vi "main.vi"(0 "Test Pins":T7, 1 "Caller Information":T8, 5 "Test Inputs":T12={"Load Current in A"=0.0, "Input Voltage in V"=[], "Nominal Output Voltage in V"=0.0, "Advance Setting"={"Prepare"={"Load SMU Output Function"=enum."VoltageSource"}, "Stimulus And Measure"={"Loop Delay in milliSecond"=1}}}, 11 "error in":errorcluster) -> (4 "Test Results":T11 {"Line Regulation in %" format="%#.5g"; "Input Voltage in V" format="%#.5g"; "Input Current in A" format="%#.5g"; "Load Current in A" format="%#.5g"; "Output Voltage in V" format="%#.5g"}, 15 "error out":errorcluster)   [LabVIEW 2020, in "LDO Line Regulation.lvlib"]
doc: "<b>Caller</b> Information is input for framework components. Mode should be set to <b>Automation</b> when running from TestStand. Sequence Context should be set to <b>ThisContext</b> when running from TestStand. The values will be updated everytime the setting is applied using \"Edit\" dialog.\n\n<b>Test Pins</b> is names of pins available in the pinmap file. Provide the right pins for the required functionality.\n\n<b>Test Inputs</b> is input required for the measurement to perform.\n\n<b>error in</b> is meant for the sequencing. <b>error in</b> should be <b>no error</b> always.\n\n<b>Test Results</b> contains all the measured data during the measurement and processed results.\n\n<b>error out</b> contains the error occured during measurement.\n\nCheck measurement documentation for more information (<Program Files>\\Soliton Technologies\\MeasurementSuite\\CodeModules\\LDO\\LDO Line Regulation.pdf)"
uses:
  LDO Line Regulation.lvlib
  Typedefs/Test Results.ctl
  Typedefs/Test Inputs.ctl
  Typedefs/Advance Settings.ctl
  Reusables/Instrument APIs/Load Output Function.ctl
  <userlib>/_Soliton/Measurement Suite/Reusables/Plugin Common/Typedefs/Caller Events.ctl
  <userlib>/_Soliton/Measurement Suite/Reusables/Plugin Common/Typedefs/Caller Information.ctl
  <userlib>/_Soliton/Measurement Suite/Reusables/Plugin Common/Typedefs/Caller Mode.ctl
  Typedefs/Test Pins.ctl
  Typedefs/Pin Dropdown.ctl
  <userlib>/_Soliton/Measurement Suite/Reusables/Plugin Common/Typedefs/Termination Monitor Info.ctl
  <vilib>/Utility/error.llb/DialogType.ctl
  dc46d5cc-eb00-4f7e-b59b-e7fbb9f2ed4c.vi
  f0cc231b-6294-4813-9d5b-a7ddc5043ff2.vi
  f8cfc4b9-01f6-4b8f-8ca0-5ef2fe22dc8a.vi
  be024a05-4f6c-4aec-bf2b-5f4e194505bf.vi
  d9360132-6dee-4b9e-876e-39170c807331.vi
  f5d431a0-41a8-4d91-8ed4-f3030fcb2f72.vi
  1f043610-9790-4767-a48a-a9d4642a4a56.vi
  bb3e62c4-a2c2-4505-9438-f842dd651d6c.vi
  ce2ee1e5-697c-4608-b941-8c9b0f21ffd9.vi
  3fc05b7f-d306-4c90-81fb-acd80905c629.vi
  34057e1b-ed15-48f4-a73e-55eccb727778.vi
  <userlib>/_Soliton/Measurement Suite/Reusables/InstrumentSessionAPIs/SessionManagerApiPath.vi
  <vilib>/Utility/sysdir.llb/Get System Directory.vi
  <vilib>/Utility/LVLibp/Get Exported File Path.vi
  <userlib>/_Soliton/Measurement Suite/Reusables/Errors/Error 6001.vi
  <userlib>/_Soliton/Measurement Suite/Reusables/Plugin Common/Plugin Common.lvlib
  <userlib>/_Soliton/Measurement Suite/Reusables/Queue Driver/Plugin Queue Driver.lvlib
panel:
  out "Progress":i32(slide) scale=-1.0..5.0
  in  "Terminate":bool
  in  "Run":bool caption="Measure"
  in  "Exit":bool
  out "Header":string
  in  "Tab Enum":T1(radio)
  out "Tab Control":T2(tab)
  in  "SystemSetup":T4={"Set Input Voltage"={"PinStatus"=0, "PinName"="", "Info"=TRUE}, "Measure Input Voltage"={"PinStatus"=0, "PinName"="", "Info"=TRUE}, "Measure Input Current"={"PinStatus"=0, "PinName"="", "Info"=TRUE}, "Set Load Current"={"PinStatus"=0, "PinName"="", "Info"=TRUE}, "Measure Output Voltage"={"PinStatus"=0, "PinName"="", "Info"=TRUE}, "Measure Load Current"={"PinStatus"=0, "PinName"="", "Info"=TRUE}}
  in  "Step Input":T5 {"Step Size (V)" min=0.0 format="%#_6p"; "Stop Value (V)" format="%#_6p"; "Start Value (V)" format="%#_6p"}
  in  "Customize Sweep Value":bool
  in  "Input Voltage (V)":dbl[](array[numeric]) format="%#_6p"
  in  "Nominal Output Voltage (V)":dbl format="%#_6p"
  in  "Customize Sweep Value":enum32{"Item 0", "Item 1"}(radio)
  in  "Load Current (A)":dbl format="%#_6p"
  in  "Advanced Settings":bool
  out "Result Tab":T6(tab)
  out "Line Regulation":cluster{"Iload (mA)":dbl[], "Vout (V)":dbl[]}(graph)
  out "Measured Values":string[][](table)
  out "Line Regulation (%/V)":dbl format="%#.3g"
  in  "Result Enum":T6(radio)
  out "Line Regulation (%)":dbl format="%#.3g"
  in  "DataLogPath":path
  in  "Caller Events":T10
  in  "ErrorOccured":errorcluster
  # "Supports NIDmmInstrument"
  # "Supports NIDmmInstrument"
  # "Supports NIDCPowerInstrument"
  # "Supports NIDCPowerInstrument"
  # "Supports NIDCPowerInstrument"
  # "Supports NIDCPowerInstrument"
  # "Fill Input Voltage list using the following"
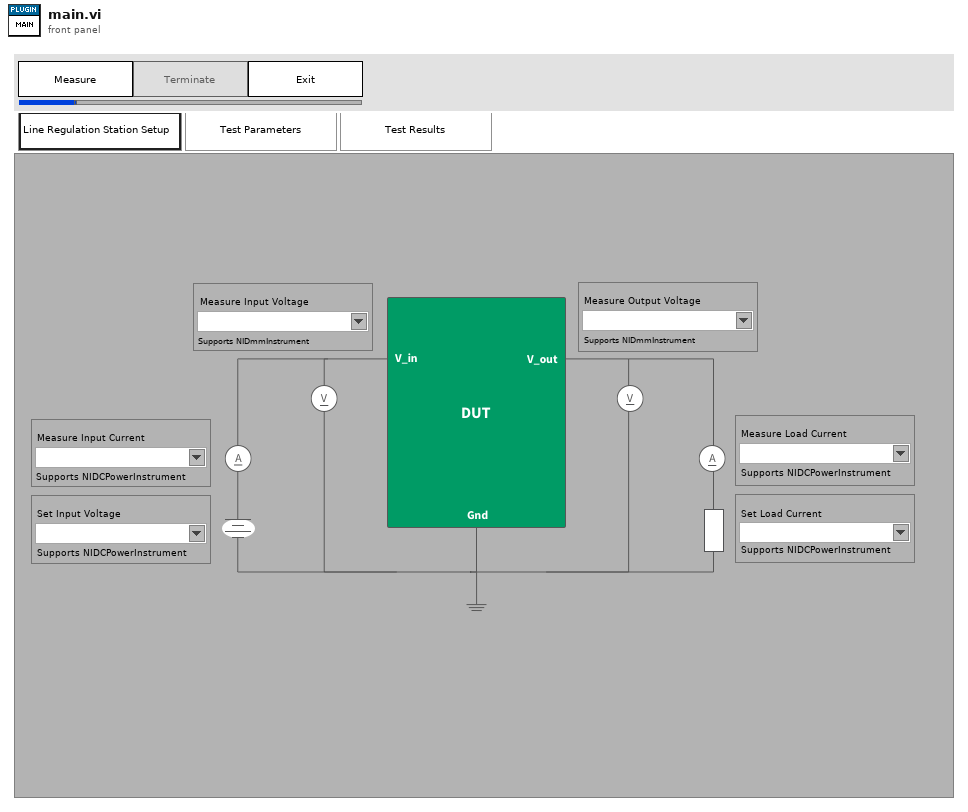
[diagram p1: front panel]
types:
  T1 = enum32{"Station Setup", "Test Parameters", "Test Results"}
  T2 = enum32{"Station Setup", "Test Parameters", "Test Results", "Debug"}
  T3 = typedef "LDO Line Regulation.lvlib/Pin Dropdown.ctl" = cluster{"PinStatus":u16, "PinName":string, "Info":bool}
  T4 = cluster{"Set Input Voltage":T3, "Measure Input Voltage":T3, "Measure Input Current":T3, "Set Load Current":T3, "Measure Output Voltage":T3, "Measure Load Current":T3}
  T5 = cluster{"Start Value (V)":dbl, "Stop Value (V)":dbl, "Step Size (V)":dbl}
  T6 = enum32{"Line Regulation Curve", "Measured Value Table View"}
  T7 = typedef "LDO Line Regulation.lvlib/Test Pins.ctl" = cluster{"Set Input Voltage":string, "Measure Input Voltage":string, "Measure Input Current":string, "Set Load Current":string, "Measure Output Voltage":string, "Measure Load Current":string}
  T8 = typedef "Plugin Common.lvlib/Caller Information.ctl" = cluster{"Mode":T9, "Sequence Context":refnum<k7>}
  T9 = typedef "Caller Mode.ctl" = enum16{"Standalone", "Automation", "MeasurementSuite"}
  T10 = typedef "Plugin Common.lvlib/Caller Events.ctl" = cluster{"Caller Event":refnum<user-event>}
  T11 = typedef "LDO Line Regulation.lvlib/Test Results.ctl" = cluster{"Input Voltage in V":dbl[], "Input Current in A":dbl[], "Output Voltage in V":dbl[], "Load Current in A":dbl[], "Line Regulation in %/V":dbl, "Line Regulation in %":dbl}
  T12 = typedef "LDO Line Regulation.lvlib/Test Inputs.ctl" = cluster{"Load Current in A":dbl, "Input Voltage in V":dbl[], "Nominal Output Voltage in V":dbl, "Advance Setting":T13}
  T13 = typedef "LDO Line Regulation.lvlib/Advance Settings.ctl" = cluster{"Prepare":cluster{"Load SMU Output Function":T14}, "Stimulus And Measure":cluster{"Loop Delay in milliSecond":u32}}
  T14 = typedef "Load Output Function.ctl" = enum16{"VoltageSource", "CurrentSource"}
  T15 = typedef "Plugin Common.lvlib/Termination Monitor Info.ctl" = cluster{"Caller Information":T8, "Execution":refnum<k7>, "Termination Monitor":refnum<k7>, "Type":string, "Plugin Name":string}
  T16 = cluster{"Termination Monitor Info":T15, "Test Inputs":T12, "Test Results":T11, "Test Results[][]":string[][], "Test Pins":T7, "Logger Folder Path":path, "Valid Logger Path?":bool, "Logger File Path":path, "UI Ctls":refnum<vi>[]}
  T17 = enum8{"Enabled", "Disabled", "Disabled and Grayed Out"}
  T18 = cluster{"Start Value":dbl, "Stop Value":dbl, "Step Size":dbl}
  T19 = cluster{"Input Voltage in V":dbl[], "Output Voltage in V":dbl[]}
  T20 = typedef "DialogType.ctl" = u16
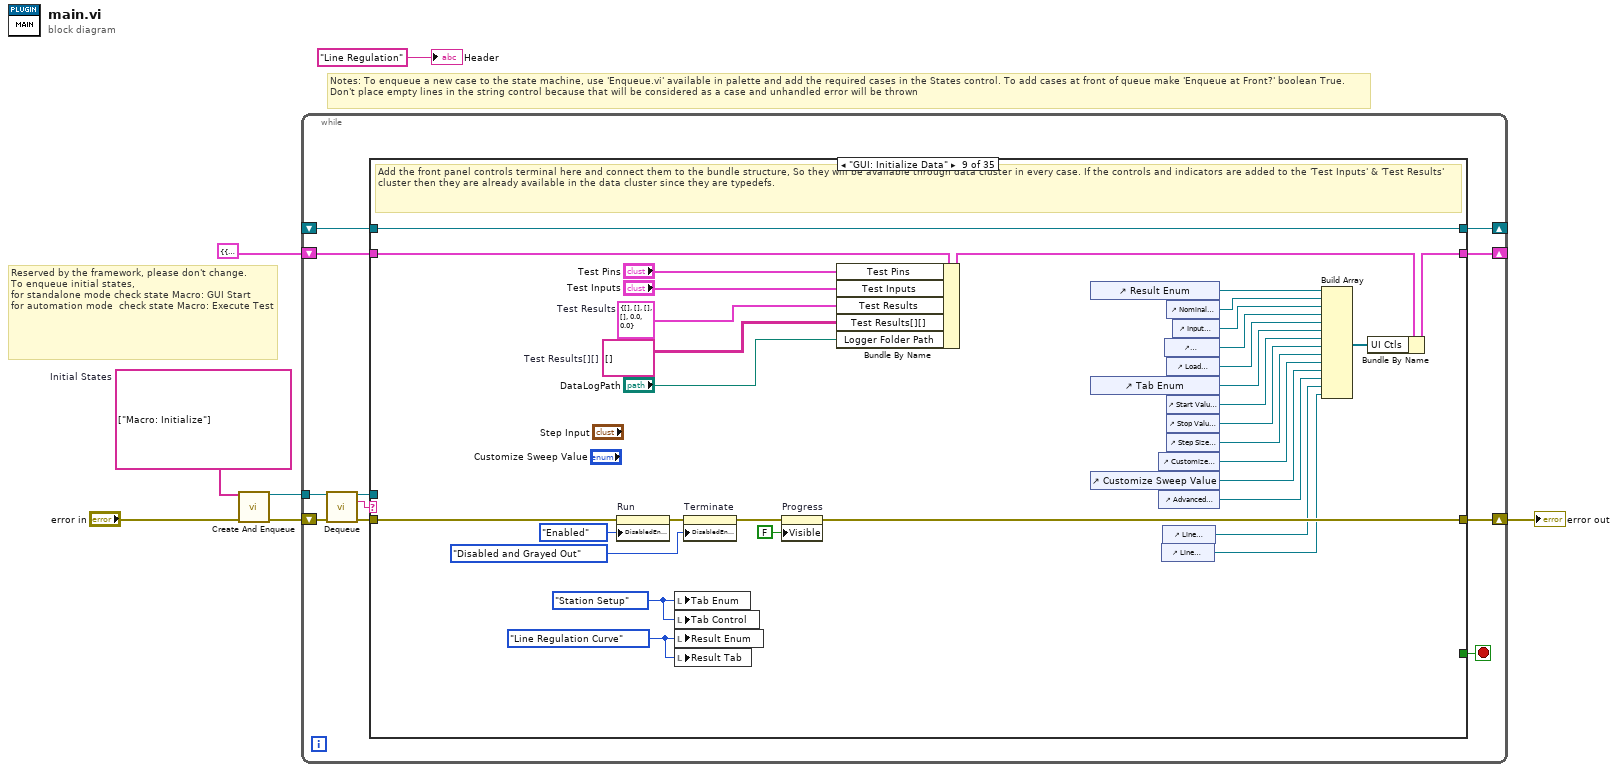
[diagram p0: block diagram]
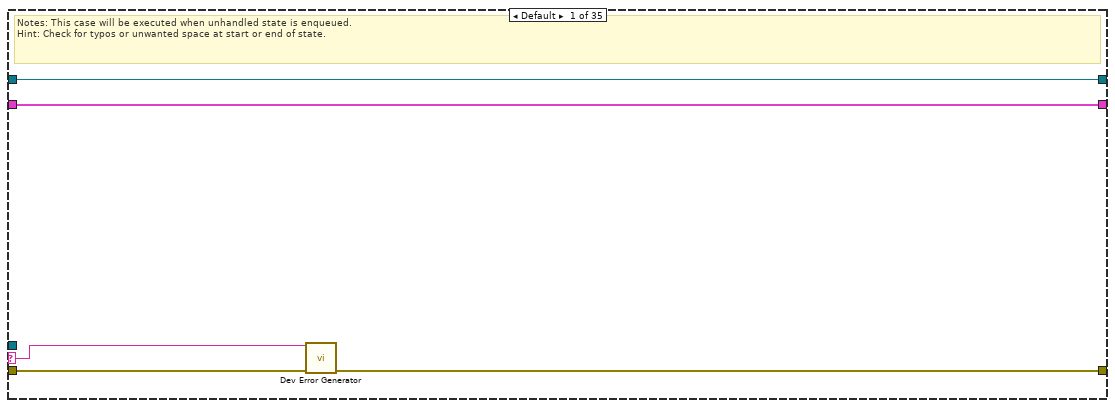
[diagram p2: hidden frame]
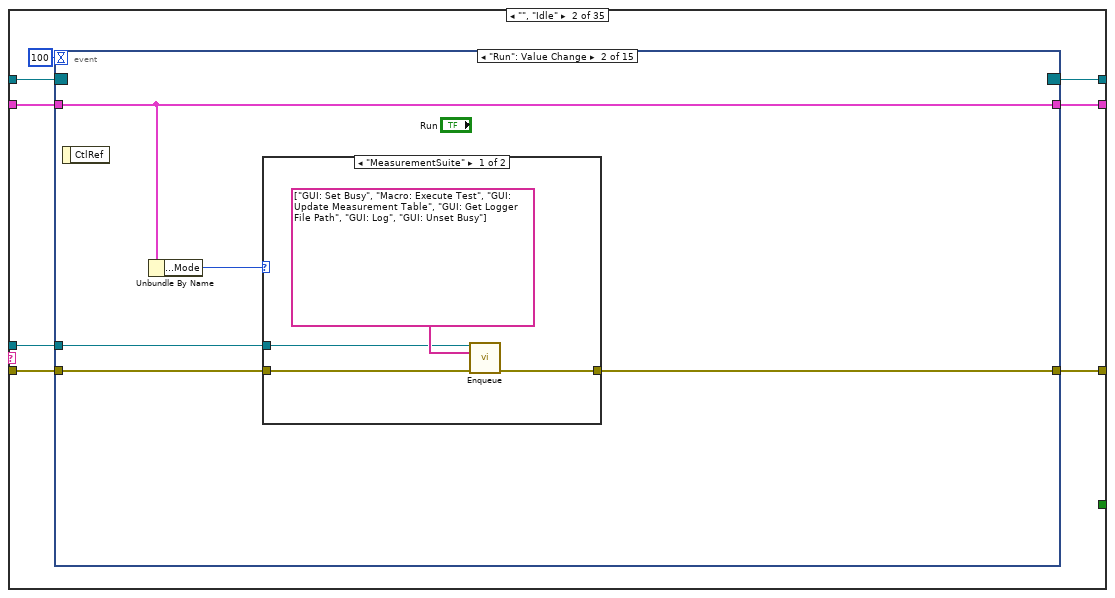
[diagram p3: hidden frame]
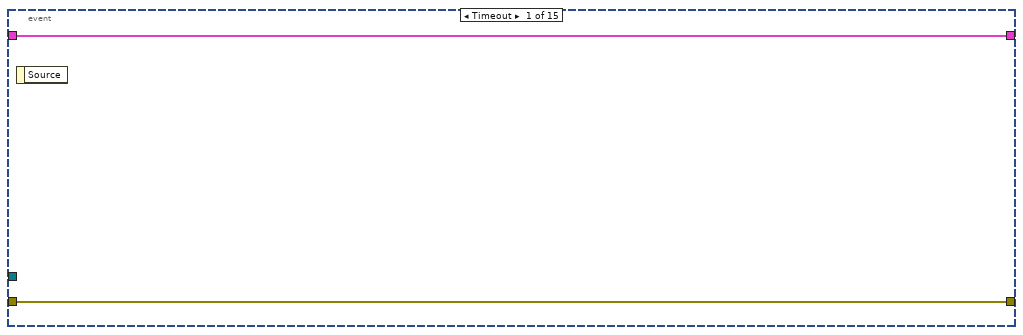
[diagram p4: hidden frame]
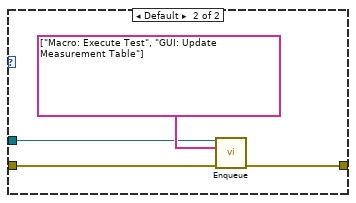
[diagram p5: hidden frame]
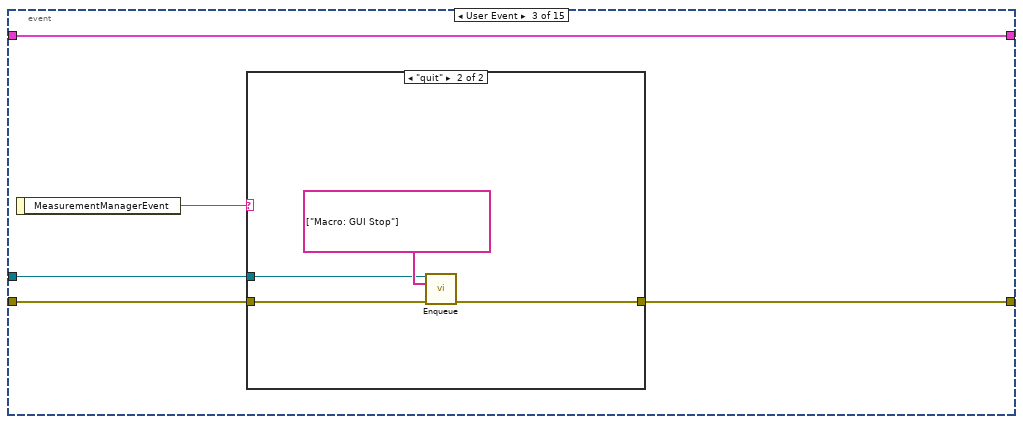
[diagram p6: hidden frame]
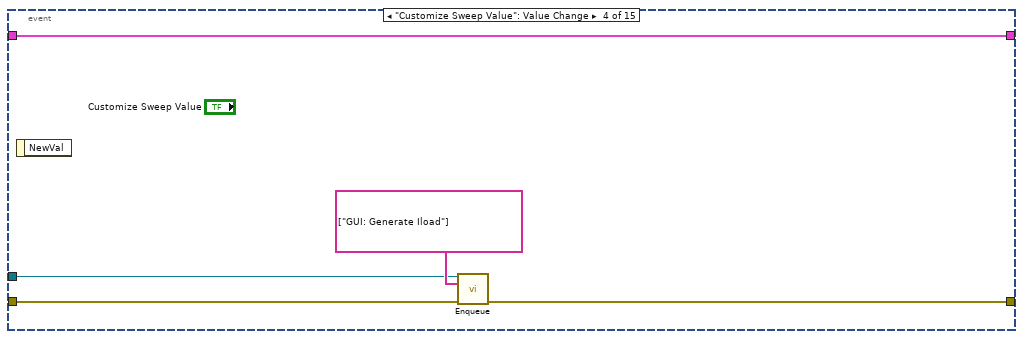
[diagram p8: hidden frame]
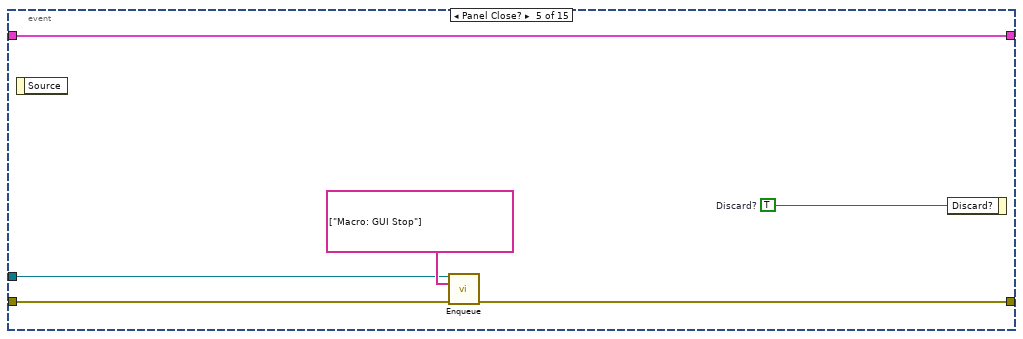
[diagram p9: hidden frame]
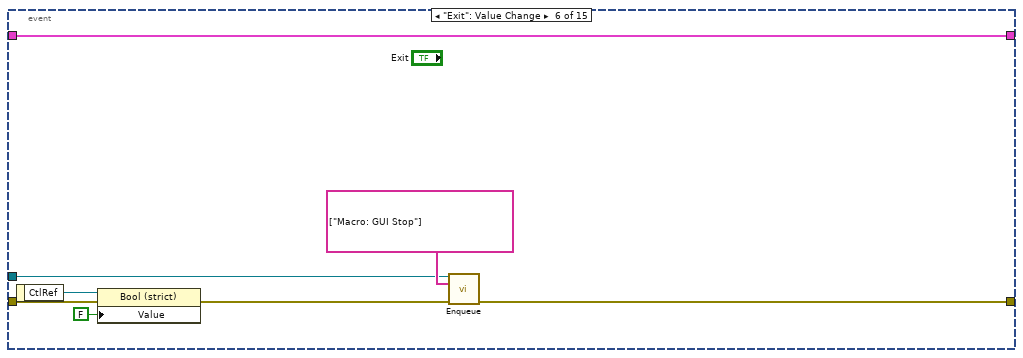
[diagram p10: hidden frame]
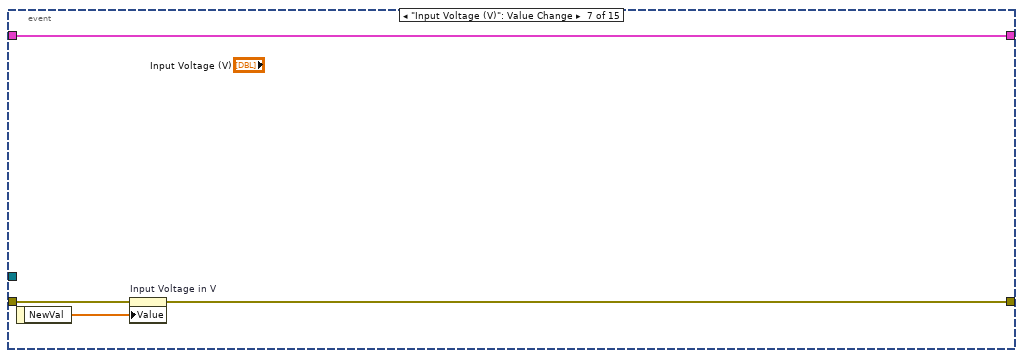
[diagram p11: hidden frame]
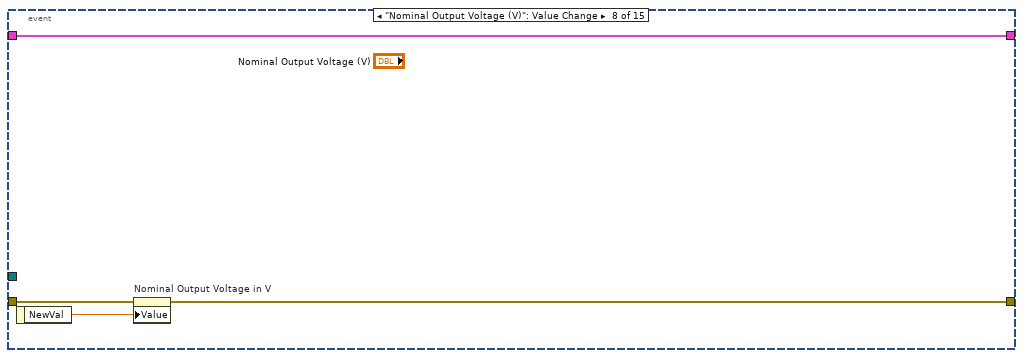
[diagram p12: hidden frame]
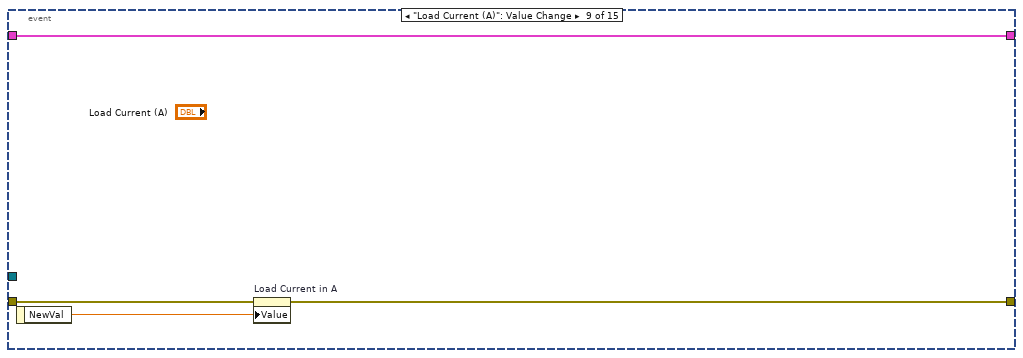
[diagram p13: hidden frame]
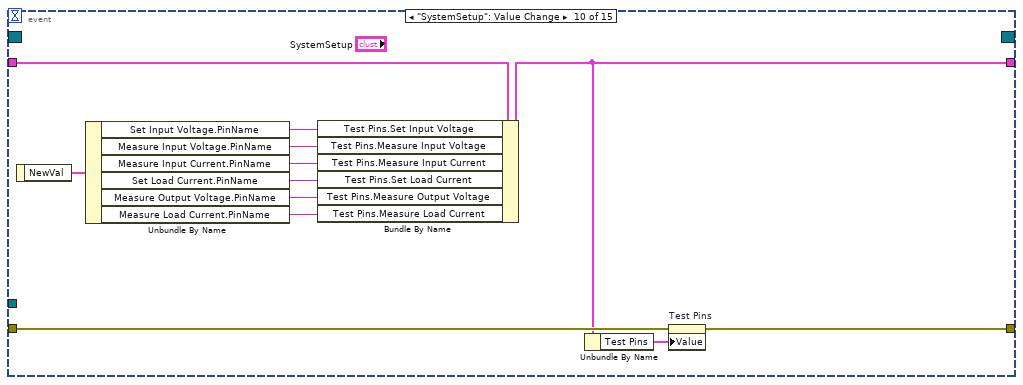
[diagram p14: hidden frame]
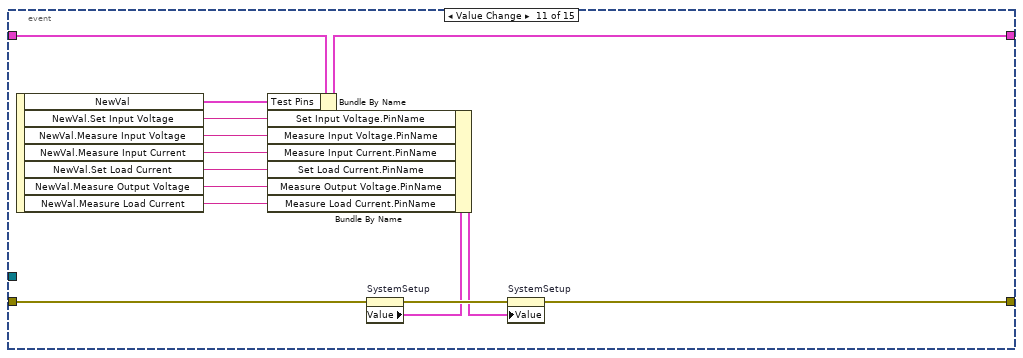
[diagram p15: hidden frame]
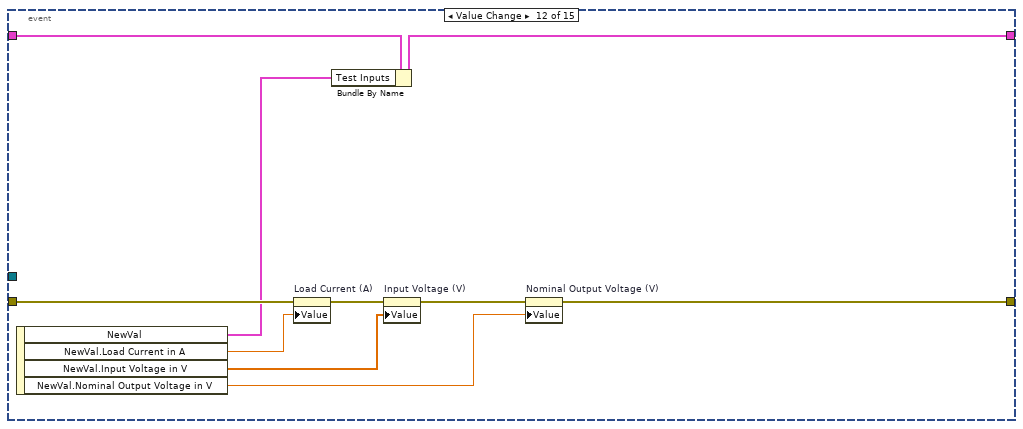
[diagram p16: hidden frame]
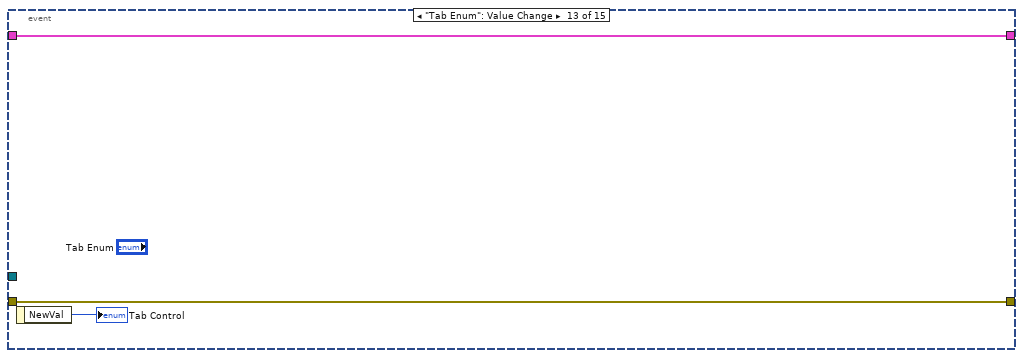
[diagram p17: hidden frame]
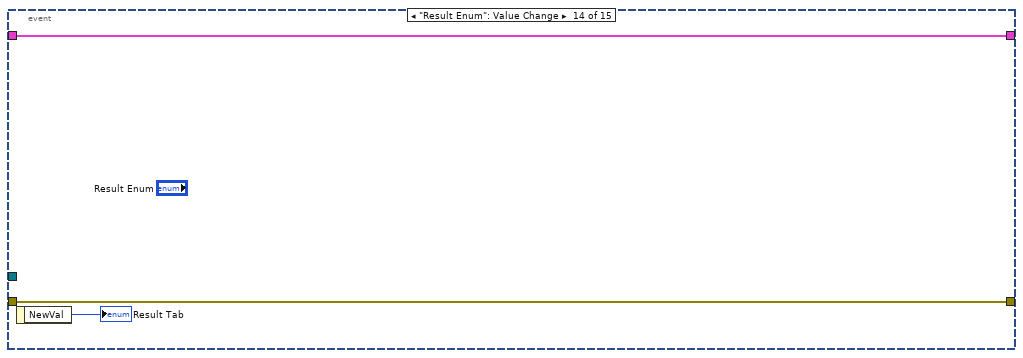
[diagram p18: hidden frame]
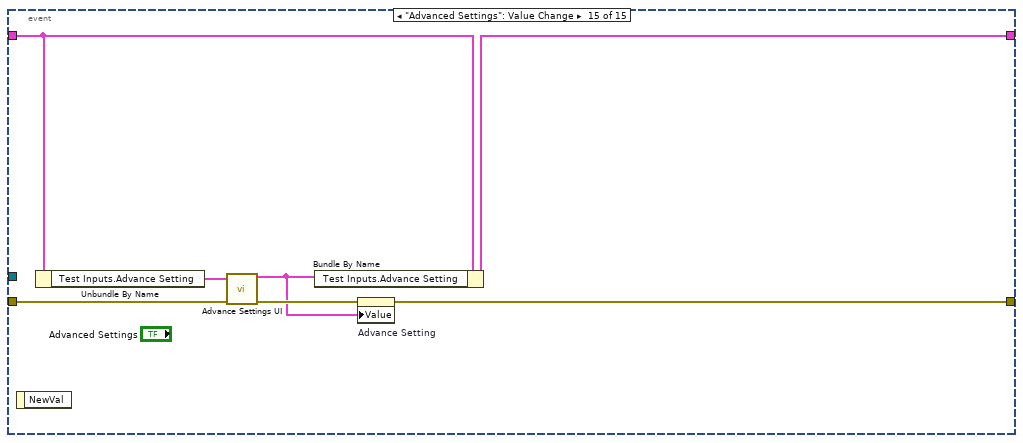
[diagram p19: hidden frame]
diagram:
  w7 = string[] ["Macro: Initialize"]  # Initial States
  # "Notes: To enqueue a new case to the state machine, use 'Enqueue.vi' available in palette and add the required cases in the States control. To add cases at front of queue make 'Enqueue at Front?' boolean True. Don't place empty lines in the string control because that will be considered as a case and unhandled error will be thrown"
  # "Reserved by the framework, please don't change. \nTo enqueue initial states,\nfor standalone mode check state Macro: GUI Start\nfor automation mode  check state Macro: Execute Test"
  n1 = call <userlib>:"Create And Enqueue.vi"("Initial States"=w7, "error in (no error)"="error in") -> ("Queue out"=w5:refnum<queue>, "error out"=w3:errorcluster)  [unwired: 12 in]
  n2 = while {
    shift-right: [w18] -> w4
    shift-left: w3 -> [w16]
    shift-right: [w14] -> _
    shift-left: T16 {"Termination Monitor Info"={"Caller Information"={"Mode"=enum."Standalone", "Sequence Context"=refnum}, "Execution"=refnum, "Termination Monitor"=refnum, "Type"="", "Plugin Name"=""}, "Test Inputs"={"Load Current in A"=0.0, "Input Voltage in V"=[], "Nominal Output Voltage in V"=0.0, "Advance Setting"={"Prepare"={"Load SMU Output Function"=enum."VoltageSource"}, "Stimulus And Measure"={"Loop Delay in milliSecond"=0}}}, "Test Results"={"Input Voltage in V"=[], "Input Current in A"=[], "Output Voltage in V"=[], "Load Current in A"=[], "Line Regulation in %/V"=0.0, "Line Regulation in %"=0.0}, "Test Results[][]"=[], "Test Pins"={"Set Input Voltage"="", "Measure Input Voltage"="", "Measure Input Current"="", "Set Load Current"="", "Measure Output Voltage"="", "Measure Load Current"=""}, "Logger Folder Path"=path "", "Valid Logger Path?"=FALSE, "Logger File Path"=path "", "UI Ctls"=[]} -> [w13]
    tunnel: w5 -> [w12]
    shift-right: [w9] -> _
    shift-left: _ -> [w10]
    stop <- w17 stop-if-true
    n3 = call <userlib>:"Dequeue.vi"("Queue in"=w12, "error in (no error)"=w16) -> ("Queue out"=w11:refnum<queue>, "Dequeued State"=w8:string, "error out"=w15:errorcluster)  [unwired: 11 in]
    n4 = case shown="\"GUI: Initialize Data\"" w8 {
      selector: w8 -> [w21 _ _ _ _ _ _ _ _ _ _ _ _ _ _ _ _ _ _ _ _ _ _ _ _ _ _ _ _ _ _ _ _ _ _]
      tunnel: w15 -> [w20 w28 w139 w148 w157 w164 w171 w176 w201 w214 w218 w221 w236 w256 w260 w277 w288 w301 w315 w320 w327 w332 w345 w358 w376 w384 w408 w458 w471 w488 w500 w506 w514 w521 w539]
      tunnel: [w22 w29 w139 w151 w158 w165 w172 w176 w199 w212 w216 w221 w230 w256 w259 w278 w289 w302 w315 w321 w328 w332 w339 w354 w369 w383 w414 w444 w463 w488 w500 w503 w514 w519 w533] -> w18
      tunnel: [_ _ _ _ _ _ _ _ _ _ _ _ _ _ _ _ _ _ _ _ _ _ _ _ _ _ _ _ _ _ _ _ _ w516 TRUE] -> w17
      tunnel: [w23 w31 w138 w141 w159 w166 w173 w175 w192 w213 w217 w220 w224 w248 w258 w279 w287 w300 w314 w319 w326 w331 w338 w359 w377 w385 w416 w460 w473 w489 w499 w511 w513 w518 w540] -> w14
      tunnel: w13 -> [w23 w30 w138 w152 w159 w166 w173 w175 w206 w213 w217 w220 w223 w247 w257 w279 w287 w300 w314 w318 w325 w331 w349 w359 w377 w385 w417 w460 w473 w490 w499 w511 w513 w518 w540]
      tunnel: w11 -> [_ w24 _ w150 w155 w162 w169 _ _ _ _ _ _ _ _ _ _ _ _ _ _ _ _ _ _ _ _ _ _ _ _ _ _ w515 w538]
      tunnel: w10 -> [w19 w26 w137 w149 w154 w161 w168 w174 w205 _ w215 w219 w237 w255 w265 w280 w295 w308 w313 w322 w329 w330 w347 w360 w379 w386 w415 w461 w474 w491 w498 w510 w512 w520 w537]
      tunnel: [w19 w25 w137 w149 w154 w161 w168 w174 w205 w211 w215 w219 w237 w255 w265 w280 w295 w308 w313 w322 w329 w330 w347 w360 w379 w386 w415 w461 w474 w491 w498 w510 w512 w520 w537] -> w9
      frame Default {
        # "Notes: This case will be executed when unhandled state is enqueued. \nHint: Check for typos or unwanted space at start or end of state."
        n5 = call <userlib>:"Dev Error Generator.vi"("State"=w21, "error in (no error)"=w20) -> ("error out"=w22:errorcluster)  [unwired: 13 in]
      }
      frame "", "Idle" {
        n6 = event shown="[1] \"Run\": Value Change" {
          selector: w26 -> [_ _ _ _ _ _ _ _ _ _ _ _ _ _ _]
          dyn-events: [_ _ _ _ _ _ _ _ _ _ _ _ _ _ _] -> w25
          timeout: 100 -> [_ _ _ _ _ _ _ _ _ _ _ _ _ _ _]
          tunnel: [w33 w35 w51 w61 w67 w75 w76 w83 w87 w89 w108 w115 w126 w129 w133] -> w31
          tunnel: w30 -> [w33 w35 w51 w61 w67 w75 w76 w83 w87 w93 w107 w114 w126 w129 w132]
          tunnel: [w32 w38 w49 w59 w64 w73 w78 w82 w86 w91 w111 w121 w125 w128 w131] -> w29
          tunnel: w28 -> [w32 w37 w50 w58 w63 w72 w79 w81 w85 w90 w113 w119 w125 w128 w135]
          tunnel: w24 -> [_ w36 w47 w57 w62 w71 _ _ _ _ _ _ _ _ _]
          event Timeout {
            n7 = event-data() -> ()  [unwired: 1 in, 1 out]
          }
          event "Run": Value Change {
            n8 = event-data() -> ()  [unwired: 1 in, 1 out]
            n9 = Unbundle By Name(w35) -> ("Termination Monitor Info.Caller Information.Mode"=w34:T9)
            n10 = case shown="\"MeasurementSuite\"" w34 {
              tunnel: [w41 w45] -> w38
              tunnel: w37 -> [w40 w44]
              tunnel: w36 -> [w39 w43]
              frame "MeasurementSuite" {
                n11 = call <userlib>:"Enqueue.vi"("Queue in"=w39, "States"=string[] ["GUI: Set Busy", "Macro: Execute Test", "GUI: Update Measurement Table", "GUI: Get Logger File Path", "GUI: Log", "GUI: Unset Busy"], "error in (no error)"=w40) -> ("error out"=w41:errorcluster)  [unwired: 11 in, 1 out]
              }
              frame Default {
                n12 = call <userlib>:"Enqueue.vi"("Queue in"=w43, "States"=string[] ["Macro: Execute Test", "GUI: Update Measurement Table"], "error in (no error)"=w44) -> ("error out"=w45:errorcluster)  [unwired: 11 in, 1 out]
              }
            }
          }
          event User Event {
            n13 = event-data() -> ("MeasurementManagerEvent"=w48:string)  [unwired: 1 in]
            n14 = case shown="\"quit\"" w48 {
              tunnel: [w52 w53] -> w49
              tunnel: w50 -> [w52 w55]
              tunnel: w47 -> [_ w54]
              frame Default {
              }
              frame "quit" {
                n15 = call <userlib>:"Enqueue.vi"("Queue in"=w54, "States"=string[] ["Macro: GUI Stop"], "error in (no error)"=w55) -> ("error out"=w53:errorcluster)  [unwired: 11 in, 1 out]
              }
            }
          }
          event "Customize Sweep Value": Value Change {
            n16 = event-data() -> ()  [unwired: 1 in, 1 out]
            n17 = call <userlib>:"Enqueue.vi"("Queue in"=w57, "States"=string[] ["GUI: Generate Iload"], "error in (no error)"=w58) -> ("error out"=w59:errorcluster)  [unwired: 11 in, 1 out]
          }
          event Panel Close? {
            w66 = TRUE  # Discard?
            n18 = event-data() -> ()  [unwired: 1 in, 1 out]
            n19 = call <userlib>:"Enqueue.vi"("Queue in"=w62, "States"=string[] ["Macro: GUI Stop"], "error in (no error)"=w63) -> ("error out"=w64:errorcluster)  [unwired: 11 in, 1 out]
            n20 = event-data("Discard?"=w66) -> ()  [unwired: 1 in, 1 out]
          }
          event "Exit": Value Change {
            n21 = event-data() -> ("CtlRef"=w69:refnum<vi>)  [unwired: 1 in]
            n22 = property class="Bool (strict)"(reference=w69, error in=w72, "Value"=FALSE) -> (error out=w70:errorcluster)  [unwired: 1 out]
            n23 = call <userlib>:"Enqueue.vi"("Queue in"=w71, "States"=string[] ["Macro: GUI Stop"], "error in (no error)"=w70) -> ("error out"=w73:errorcluster)  [unwired: 11 in, 1 out]
          }
          event "Input Voltage (V)": Value Change {
            n24 = event-data() -> ("NewVal"=w77:dbl[])  [unwired: 1 in]
            n25 = property on="Input Voltage in V" class="Arr (strict)"(error in=w79, "Value"=w77) -> (error out=w78:errorcluster)  [unwired: 1 in, 1 out]
          }
          event "Nominal Output Voltage (V)": Value Change {
            n26 = event-data() -> ("NewVal"=w80:dbl)  [unwired: 1 in]
            n27 = property on="Nominal Output Voltage in V" class="DigNum (strict)"(error in=w81, "Value"=w80) -> (error out=w82:errorcluster)  [unwired: 1 in, 1 out]
          }
          event "Load Current (A)": Value Change {
            n28 = event-data() -> ("NewVal"=w84:dbl)  [unwired: 1 in]
            n29 = property on="Load Current in A" class="DigNum (strict)"(error in=w85, "Value"=w84) -> (error out=w86:errorcluster)  [unwired: 1 in, 1 out]
          }
          event "SystemSetup": Value Change {
            n30 = event-data() -> ("NewVal"=w92:T4)  [unwired: 1 in]
            n31 = Unbundle By Name(w92) -> ("Set Input Voltage.PinName"=w99:string, "Measure Input Voltage.PinName"=w98:string, "Measure Input Current.PinName"=w97:string, "Set Load Current.PinName"=w96:string, "Measure Output Voltage.PinName"=w95:string, "Measure Load Current.PinName"=w94:string)
            n32 = Bundle By Name(cluster=w93, "Test Pins.Set Input Voltage"=w99, "Test Pins.Measure Input Voltage"=w98, "Test Pins.Measure Input Current"=w97, "Test Pins.Set Load Current"=w96, "Test Pins.Measure Output Voltage"=w95, "Test Pins.Measure Load Current"=w94) -> (w89:T16)
            n33 = Unbundle By Name(w89) -> ("Test Pins"=w88:T7)
            n34 = property on="Test Pins" class="Clust (strict)"(error in=w90, "Value"=w88) -> (error out=w91:errorcluster)  [unwired: 1 in, 1 out]
          }
          event Value Change {
            n35 = event-data() -> ("NewVal"=w100:T7, "NewVal.Set Input Voltage"=w106:string, "NewVal.Measure Input Voltage"=w105:string, "NewVal.Measure Input Current"=w104:string, "NewVal.Set Load Current"=w103:string, "NewVal.Measure Output Voltage"=w102:string, "NewVal.Measure Load Current"=w101:string)  [unwired: 1 in]
            n36 = Bundle By Name(cluster=w107, "Test Pins"=w100) -> (w108:T16)
            n37 = property on="SystemSetup" class="Clust (strict)"(error in=w113) -> (error out=w112:errorcluster, "Value"=w110:T4)  [unwired: 1 in, 1 out]
            n38 = Bundle By Name(cluster=w110, "Set Input Voltage.PinName"=w106, "Measure Input Voltage.PinName"=w105, "Measure Input Current.PinName"=w104, "Set Load Current.PinName"=w103, "Measure Output Voltage.PinName"=w102, "Measure Load Current.PinName"=w101) -> (w109:T4)
            n39 = property on="SystemSetup" class="Clust (strict)"(error in=w112, "Value"=w109) -> (error out=w111:errorcluster)  [unwired: 1 in, 1 out]
          }
          event Value Change {
            n40 = event-data() -> ("NewVal"=w116:T12, "NewVal.Load Current in A"=w117:dbl, "NewVal.Input Voltage in V"=w122:dbl[], "NewVal.Nominal Output Voltage in V"=w120:dbl)  [unwired: 1 in]
            n41 = property on="Load Current (A)" class="DigNum (strict)"(error in=w119, "Value"=w117) -> (error out=w118:errorcluster)  [unwired: 1 in, 1 out]
            n42 = Bundle By Name(cluster=w114, "Test Inputs"=w116) -> (w115:T16)
            n43 = property on="Input Voltage (V)" class="Arr (strict)"(error in=w118, "Value"=w122) -> (error out=w123:errorcluster)  [unwired: 1 in, 1 out]
            n44 = property on="Nominal Output Voltage (V)" class="DigNum (strict)"(error in=w123, "Value"=w120) -> (error out=w121:errorcluster)  [unwired: 1 in, 1 out]
          }
          event "Tab Enum": Value Change {
            n45 = event-data() -> ("NewVal"=→"Tab Control":T1)  [unwired: 1 in]
          }
          event "Result Enum": Value Change {
            n46 = event-data() -> ("NewVal"=→"Result Tab":T6)  [unwired: 1 in]
          }
          event "Advanced Settings": Value Change {
            n47 = event-data() -> ()  [unwired: 1 in, 1 out]
            n48 = Unbundle By Name(w132) -> ("Test Inputs.Advance Setting"=w134:T13)
            n49 = call "Advance Settings UI.vi"("Advance Setting"=w134, "error in (no error)"=w135) -> ("Advance Setting Out"=w130:T13, "error out"=w136:errorcluster)  [unwired: 12 in]
            n50 = Bundle By Name(cluster=w132, "Test Inputs.Advance Setting"=w130) -> (w133:T16)
            n51 = property on="Advance Setting" class="Clust (strict)"(error in=w136, "Value"=w130) -> (error out=w131:errorcluster)  [unwired: 1 in, 1 out]
          }
        }
      }
      frame "----------------- Macro ---------------" {
        # "Not used. category splitter"
      }
      frame "Macro: Initialize" {
        w145 = string[] ["Macro: GUI Start"]  # Standalone: Start the debug
        w146 = string[] ["Macro: Execute Test", "Exit"]  # Automation: Execute and stop
        # "Hidden in UI"
        # "This case decides the mode of the execution. Debug Mode: The plugin will act as a standalone GUI where user can change inputs, run test and debug the system. automation mode: The plugin will act as a flat code and go through all the test procedures and stops."
        n52 = call <userlib>:"Get Mode.vi"("Caller Information"="Caller Information", "error in (no error)"=w148) -> ("Automation(F) \\ Standalone (T)"=w144:bool, "error out"=w147:errorcluster)  [unwired: 12 in]
        n53 = Bundle By Name(cluster=w152, "Termination Monitor Info.Caller Information"="Caller Information") -> (w141:T16)
        n54 = Select(t=w145, s=w144, f=w146) -> (s? t:f=w143:string[])
        n55 = call <userlib>:"Enqueue.vi"("Queue in"=w150, "States"=w143, "Enqueue at Front?(F)"=TRUE, "error in (no error)"=w147) -> ("error out"=w151:errorcluster)  [unwired: 10 in, 1 out]
      }
      frame "Macro: Execute Test" {
        w156 = string[] ["TerminationMonitor: Start", "Test: Start", "Test: Prepare DCPower", "Test: Prepare DMM", "Test: Set Load Current", "Test: Sweep Over Voltage", "Test: Cleanup DCPower", "Test: Cleanup DMM", "Test: Calculate Load", "Test: Update UI", "Test: End", "TerminationMonitor: Stop"]  # Test Procedure
        # "List the states required for the test procedure. This state will be called in both automation mode and standalone mode when requested to run the test.\nDont remove 'Test: Start' and 'Test: End'."
        n56 = call <userlib>:"Enqueue.vi"("Queue in"=w155, "States"=w156, "Enqueue at Front?(F)"=TRUE, "error in (no error)"=w157) -> ("error out"=w158:errorcluster)  [unwired: 10 in, 1 out]
      }
      frame "Macro: GUI Start" {
        # "Initialize the data cluster for the standalone mode and register for the event from caller.\nDon't remove 'GUI: Initialize Data' and 'GUI: Register Event'."
        n57 = call <userlib>:"Enqueue.vi"("Queue in"=w162, "States"=string[] ["GUI: Initialize Data", "GUI: Register Event"], "Enqueue at Front?(F)"=TRUE, "error in (no error)"=w164) -> ("error out"=w165:errorcluster)  [unwired: 10 in, 1 out]
      }
      frame "Macro: GUI Stop" {
        # "Cleanups the standalone mode and stop the execution.\nDon't remove 'GUI: Unregister Event', 'GUI: Cleanup Data' and 'Exit'."
        n58 = call <userlib>:"Enqueue.vi"("Queue in"=w169, "States"=string[] ["GUI: Unregister Event", "GUI: Cleanup Data", "Exit"], "Enqueue at Front?(F)"=TRUE, "error in (no error)"=w171) -> ("error out"=w172:errorcluster)  [unwired: 10 in, 1 out]
      }
      frame "--------------- GUI Mode-----------------" {
        # "Not used. category splitter"
      }
      frame "GUI: Initialize Data" {
        w193 = T6."Line Regulation Curve" ("Result Enum")
        w194 = T1."Station Setup" ("Tab Enum")
        w197 = string[][] []  # Test Results[][]
        w208 = T11 {"Input Voltage in V"=[], "Input Current in A"=[], "Output Voltage in V"=[], "Load Current in A"=[], "Line Regulation in %/V"=0.0, "Line Regulation in %"=0.0}  # Test Results
        # "Add the front panel controls terminal here and connect them to the bundle structure, So they will be available through data cluster in every case. If the controls and indicators are added to the 'Test Inputs' & 'Test Results' cluster then they are already available in the data cluster since they are typedefs."
        n59 = property on="Run" class="Bool (strict)"(error in=w201, "DisabledEnum"=T17."Enabled" ("Disabled")) -> (error out=w204:errorcluster)  [unwired: 1 in, 1 out]
        n60 = local write "Tab Enum"(w194) -> ()
        n61 = local write "Tab Control"(w194) -> ()
        n62 = local write "Result Enum"(w193) -> ()
        n63 = local write "Result Tab"(w193) -> ()
        n64 = property on="Terminate" class="Bool (strict)"(error in=w204, "DisabledEnum"=T17."Disabled and Grayed Out" ("Disabled")) -> (error out=w200:errorcluster)  [unwired: 1 in, 1 out]
        n65 = property on="Progress" class="Slide (strict)"(error in=w200, "Visible"=FALSE) -> (error out=w199:errorcluster)  [unwired: 1 in, 1 out]
        n66 = Bundle By Name(cluster=w206, "Test Pins"="Test Pins", "Test Inputs"="Test Inputs", "Test Results"=w208, "Test Results[][]"=w197, "Logger Folder Path"="DataLogPath") -> (w207:T16)
        n67 = control-ref of="Result Enum"() -> (w191:refnum<vi>)
        n68 = control-ref of="Tab Enum"() -> (w186:refnum<vi>)
        n69 = control-ref of="Customize Sweep Value"() -> (w181:refnum<vi>)
        n70 = control-ref of="Customize Sweep Value"() -> (w182:refnum<vi>)
        n71 = control-ref of="Advanced Settings"() -> (w180:refnum<vi>)
        n72 = control-ref of="Line Regulation (%)"() -> (w177:refnum<vi>)
        n73 = control-ref of="Line Regulation (%/V)"() -> (w178:refnum<vi>)
        n74 = control-ref of="SystemSetup"() -> (w188:refnum<vi>)
        n75 = control-ref of="Nominal Output Voltage (V)"() -> (w190:refnum<vi>)
        n76 = control-ref of="Load Current (A)"() -> (w187:refnum<vi>)
        n77 = control-ref of="Start Value (V)"() -> (w185:refnum<vi>)
        n78 = control-ref of="Stop Value (V)"() -> (w184:refnum<vi>)
        n79 = control-ref of="Step Size (V)"() -> (w183:refnum<vi>)
        n80 = control-ref of="Input Voltage (V)"() -> (w189:refnum<vi>)
        n81 = Build Array(w191, w190, w189, w188, w187, w186, w185, w184, w183, w182, w181, w180, w178, w177) -> (w179:refnum<vi>[])
        n82 = Bundle By Name(cluster=w207, "UI Ctls"=w179) -> (w192:T16)
      }
      frame "GUI: Register Event" {
        # "Hidden in UI"
        # "Register for the events from caller."
        n83 = register-events(error in=w214, "Caller Events") -> (reference out=w211:refnum<event-registration>, error out=w212:errorcluster)  [unwired: 1 in]
      }
      frame "GUI: Unregister Event" {
        n84 = Unregister For Events(event registration refnum=w215, error in=w218) -> (error out=w216:errorcluster)
      }
      frame "GUI: Cleanup Data" {
        # "Cleanup the reference or other resources before exiting"
      }
      frame "GUI: Generate Iload" {
        n85 = property on="Step Input" class="Clust (strict)"(error in=w236) -> (error out=w225:errorcluster, "Value"=w235:T18)  [unwired: 1 in, 1 out]
        n86 = Unbundle By Name(w235) -> ("Start Value"=w234:dbl, "Stop Value"=w233:dbl, "Step Size"=w232:dbl)
        n87 = property on="Customize Sweep Value" class="RadioBtnsControl (strict)"(error in=w225) -> (error out=w227:errorcluster, "Value"=w229:enum32{"Item 0", "Item 1"})  [unwired: 1 in, 1 out]
        n88 = call "Get Range Values[].vi"("Start"=w234, "Stop"=w233, "Step Size"=w232) -> ("Values[]"=w228:dbl[])  [unwired: 12 in]
        n89 = case shown="\"Item 1\"" w229 {
          tunnel: w228 -> [w239 w240]
          tunnel: [w239 w242] -> w222
          tunnel: w227 -> [w238 w244]
          tunnel: [w238 w243] -> w226
          frame "Item 0", Default {
            # "Replace Existing"
          }
          frame "Item 1" {
            # "Append to end"
            n90 = property on="Input Voltage (V)" class="Arr (strict)"(error in=w244) -> (error out=w243:errorcluster, "Value"=w241:dbl[])  [unwired: 1 in, 1 out]
            n91 = Insert Into Array(array=w241, new element=w240) -> (w242:dbl[])  [unwired: 1 in]
          }
        }
        n92 = property on="Input Voltage (V)" class="Arr (strict)"(error in=w226, "Value"=w222) -> (error out=w231:errorcluster)  [unwired: 1 in, 1 out]
        n93 = Bundle By Name(cluster=w223, "Test Inputs.Input Voltage in V"=w222) -> (w224:T16)
        n94 = property on="Input Voltage in V" class="Arr (strict)"(error in=w231, "Value"=w222) -> (error out=w230:errorcluster)  [unwired: 1 in, 1 out]
      }
      frame "GUI: Update Measurement Table" {
        n95 = Unbundle By Name(w247) -> ("Test Results.Input Voltage in V"=w254:dbl[], "Test Results.Input Current in A"=w253:dbl[], "Test Results.Output Voltage in V"=w251:dbl[], "Test Results.Load Current in A"=w250:dbl[])
        n96 = Build Array(w254, w253, w251, w250) -> (w252:dbl[][])
        n97 = Transpose 2D Array(2D array=w252) -> (transposed array=w249:dbl[][])
        n98 = Number To Fractional String(number=w249, precision (6)=i16 5) -> (F-format string=w246:string[][])  [unwired: 2 in]
        "Measured Values" <- w246
        n99 = Bundle By Name(cluster=w247, "Test Results[][]"=w246) -> (w248:T16)
      }
      frame "GUI: Get Logger File Path" {
        n100 = Unbundle By Name(w257) -> ("Logger Folder Path"=w264:path)
        n101 = call <vilib>:"Check if File or Folder Exists.vi"("error in (no error)"=w260, "path"=w264) -> ("error out"=w263:errorcluster, "file or folder exists?"=w262:bool, "dup path"=w261:path)  [unwired: 7 in]
        n102 = case shown="True" w262 {
          tunnel: [w267 w269] -> w259
          tunnel: w263 -> [w267 w269]
          tunnel: w257 -> [w266 w272]
          tunnel: [w266 w271] -> w258
          tunnel: w261 -> [_ w268]
          frame False {
          }
          frame True {
            n103 = Bundle By Name(cluster=w272, "Valid Logger Path?"=TRUE ("Valid Logger path?"), "Logger File Path"=w268) -> (w271:T16)
          }
        }
      }
      frame "GUI: Log" {
        n104 = Unbundle By Name(w279) -> ("Valid Logger Path?"=w273:bool, "Test Inputs"=w275:T12, "Test Results"=w276:T11, "Logger File Path"=w274:path)
        n105 = case shown="True" w273 {
          tunnel: [w281 w286] -> w278
          tunnel: w277 -> [w281 w285]
          tunnel: w276 -> [_ w284]
          tunnel: w275 -> [_ w283]
          tunnel: w274 -> [_ w282]
          frame False {
          }
          frame True {
            n106 = call "Log Data.vi"("Test Inputs"=w283, "Test Results"=w284, "DataLogger File Path"=w282, "error in (no error)"=w285) -> ("error out"=w286:errorcluster)  [unwired: 11 in]
          }
        }
      }
      frame "GUI: Set Busy" {
        n107 = Unbundle By Name(w287) -> ("UI Ctls"=w293:refnum<vi>[])
        n108 = for {
          tunnel: [w298] -> w294 mode=indexing
          tunnel: w288 -> [w299]
          tunnel: w293 -> [w297] mode=indexing
          tunnel: T17."Disabled and Grayed Out" ("Disabled") -> [w296]
          n109 = property class="Ctl"(reference=w297, error in=w299, "DisabledEnum"=w296) -> (error out=w298:errorcluster)  [unwired: 1 out]
        }
        n110 = Merge Errors(w294) -> (w291:errorcluster)
        n111 = call "Defer Front Panel.vi"("Defer Front Panel?"=TRUE, "error in"=w291) -> ("error out"=w289:errorcluster)  [unwired: 13 in]
      }
      frame "GUI: Unset Busy" {
        n112 = Unbundle By Name(w300) -> ("UI Ctls"=w306:refnum<vi>[])
        n113 = for {
          tunnel: [w311] -> w307 mode=indexing
          tunnel: w301 -> [w312]
          tunnel: w306 -> [w310] mode=indexing
          tunnel: T17."Enabled" ("Disabled") -> [w309]
          n114 = property class="Ctl"(reference=w310, error in=w312, "DisabledEnum"=w309) -> (error out=w311:errorcluster)  [unwired: 1 out]
        }
        n115 = Merge Errors(w307) -> (w304:errorcluster)
        n116 = call "Defer Front Panel.vi"("Defer Front Panel?"=FALSE, "error in"=w304) -> ("error out"=w302:errorcluster)  [unwired: 13 in]
      }
      frame "------------ TerminationMonitor -----------" {
        # "Not used. category splitter"
      }
      frame "TerminationMonitor: Start" {
        # "Termination Monitor monitors the execution of the caller. Use Termination Monitor Status to get the termination status. If the caller is terminating, stop the test procedure, cleanup and stop."
        n117 = Unbundle By Name(w318) -> ("Termination Monitor Info.Caller Information"=w317:T8)
        n118 = call <userlib>:"Termination Monitor Start.vi"("Caller Information"=w317, "error in (no error)"=w320) -> ("Termination Monitor Info out"=w316:T15, "error out"=w321:errorcluster)  [unwired: 12 in]
        n119 = Bundle By Name(cluster=w318, "Termination Monitor Info"=w316) -> (w319:T16)
      }
      frame "TerminationMonitor: Stop" {
        n120 = Unbundle By Name(w325) -> ("Termination Monitor Info"=w324:T15)
        n121 = call <userlib>:"Termination Monitor Stop.vi"("Status Info in"=w324, "error in (no error)"=w327) -> ("Status Info out"=w323:T15, "error out"=w328:errorcluster)  [unwired: 12 in]
        n122 = Bundle By Name(cluster=w325, "Termination Monitor Info"=w323) -> (w326:T16)
      }
      frame "------------ Automation Mode -----------" {
        # "Not used. category splitter"
      }
      frame "Test: Start" {
        # "Reinitialize/Reset/Update the data from the UI to the data cluster so that the data will be considered for the test procedure.\nReset the Test Results."
        n123 = local read "DataLogPath"() -> (w333:path)
        n124 = local read "Test Inputs"() -> (w348:T12)
        n125 = local read "Test Pins"() -> (w334:T7)
        n126 = property on="Run" class="Bool (strict)"(error in=w345, "DisabledEnum"=T17."Disabled and Grayed Out" ("Disabled")) -> (error out=w343:errorcluster)  [unwired: 1 in, 1 out]
        n127 = Bundle By Name(cluster=w349, "Test Pins"=w334, "Test Inputs"=w348, "Test Results"=T11 {"Input Voltage in V"=[], "Input Current in A"=[], "Output Voltage in V"=[], "Load Current in A"=[], "Line Regulation in %/V"=0.0, "Line Regulation in %"=0.0}, "Logger Folder Path"=w333) -> (w338:T16)
        n128 = property on="Terminate" class="Bool (strict)"(error in=w343, "DisabledEnum"=T17."Enabled" ("Disabled")) -> (error out=w340:errorcluster)  [unwired: 1 in, 1 out]
        n129 = Unbundle By Name(w338) -> ("Test Inputs.Input Voltage in V"=w337:dbl[])
        n130 = Array Size(array=w337) -> (size(s)=w336:i32)
        n131 = property on="Progress" class="Slide (strict)"(error in=w340, "Visible"=TRUE, "Scale.Maximum"=w336, "Value"=0 ("Progress")) -> (error out=w339:errorcluster)  [unwired: 1 in, 1 out]
      }
      frame "Test: Prepare DCPower" {
        # "Set load current as Initial current\nSet first index of Input Voltage as initial Voltage"
        n132 = Unbundle By Name(w359) -> ("Test Pins.Set Load Current"=w353:string, "Test Inputs.Load Current in A"=w352:dbl, "Test Inputs.Advance Setting.Prepare.Load SMU Output Function"=w351:T14, "Test Pins.Set Input Voltage"=w357:string, "Test Inputs.Input Voltage in V"=w356:dbl[])
        n133 = Index Array(array=w356) -> (element=w350:dbl)  [unwired: 1 in]
        n134 = call "Prepare Source.vi"("Set Vin"=w357, "Initial Voltage Level (V)"=w350, "error in (no error)"=w358) -> ("error out"=w355:errorcluster)  [unwired: 12 in]
        n135 = call "Prepare Load.vi"("PinName"=w353, "Load Current Level (A)"=w352, "error in (no error)"=w355, "Load Output Function"=w351) -> ("error out"=w354:errorcluster)  [unwired: 11 in]
      }
      frame "Test: Prepare DMM" {
        w373 = 1 items=["DC Volts"=1, "AC Volts"=2, "DC Current"=3, "AC Current"=4, "2-Wire Resistance"=5, "4-Wire Resistance"=101, "Frequency"=104, "Period"=105, "AC Volts DC Coupled"=1001, "Diode"=1002, "Waveform Voltage"=1003, "Waveform Current"=1004, "Capacitance"=1005, "Inductance"=1006, "Temperature"=108] ("Configuration:Function")
        w374 = 1 items=["DC Volts"=1, "AC Volts"=2, "DC Current"=3, "AC Current"=4, "2-Wire Resistance"=5, "4-Wire Resistance"=101, "Frequency"=104, "Period"=105, "AC Volts DC Coupled"=1001, "Diode"=1002, "Waveform Voltage"=1003, "Waveform Current"=1004, "Capacitance"=1005, "Inductance"=1006, "Temperature"=108] ("Configuration:Function")
        # "Adding Abort.vi to stop prev acquisition"
        n136 = Unbundle By Name(w377) -> ("Test Pins.Measure Input Voltage"=w367:string, "Test Pins.Measure Output Voltage"=w368:string)
        n137 = call "Pin Name to Reference.vim"("Pin Name"=w368, "type"=refnum<k15> refnum ("instrument handle"), "error in (no error)"=w376) -> ("Reference"=w365:refnum<k15>, "error out"=w375:errorcluster)  [unwired: 7 in, 4 out]
        n138 = call <instrlib>:"niDMM Abort.vi"("error in (no error)"=w375, "instrument handle"=w365) -> ("error out"=w366:errorcluster, "instrument handle out"=w364:refnum<k15>)  [unwired: 8 in]
        n139 = property class="niDMM"(reference=w364, error in=w366, "Function"=w374) -> (error out=w370:errorcluster)  [unwired: 1 out]
        n140 = call "Pin Name to Reference.vim"("Pin Name"=w367, "type"=refnum<k15> refnum ("instrument handle"), "error in (no error)"=w370) -> ("Reference"=w362:refnum<k15>, "error out"=w372:errorcluster)  [unwired: 7 in, 4 out]
        n141 = call <instrlib>:"niDMM Abort.vi"("error in (no error)"=w372, "instrument handle"=w362) -> ("error out"=w363:errorcluster, "instrument handle out"=w361:refnum<k15>)  [unwired: 8 in]
        n142 = property class="niDMM"(reference=w361, error in=w363, "Function"=w373) -> (error out=w369:errorcluster)  [unwired: 1 out]
      }
      frame "Test: Set Load Current" {
        n143 = Unbundle By Name(w385) -> ("Test Pins.Set Load Current"=w382:string, "Test Inputs.Load Current in A"=w381:dbl, "Test Inputs.Advance Setting.Prepare.Load SMU Output Function"=w380:T14)
        n144 = call "Set Load Current.vi"("PinName"=w382, "current level"=w381, "error in (no error)"=w384, "OutputFunction"=w380) -> ("error out"=w383:errorcluster)  [unwired: 11 in]
      }
      frame "Test: Sweep Over Voltage" {
        n145 = Unbundle By Name(w417) -> ("Termination Monitor Info"=w413:T15, "Test Inputs.Advance Setting.Stimulus And Measure.Loop Delay in milliSecond"=w391:u32, "Test Pins.Set Input Voltage"=w390:string, "Test Inputs.Input Voltage in V"=w388:dbl[], "Test Pins.Measure Input Current"=w398:string, "Test Pins.Measure Load Current"=w399:string, "Test Pins.Measure Input Voltage"=w400:string, "Test Pins.Measure Output Voltage"=w401:string)
        n146 = call "Pin Name to Reference.vim"("Pin Name"=w401, "type"=refnum<k15> refnum ("instrument handle"), "error in (no error)"=w408) -> ("Reference"=w394:refnum<k15>, "error out"=w404:errorcluster)  [unwired: 7 in, 4 out]
        n147 = call "Pin Name to Reference.vim"("Pin Name"=w400, "type"=refnum<k15> refnum ("instrument handle"), "error in (no error)"=w404) -> ("Reference"=w395:refnum<k15>, "error out"=w403:errorcluster)  [unwired: 7 in, 4 out]
        n148 = call "Pin Name to Reference.vim"("Pin Name"=w399, "type"=refnum<k15> refnum ("instrument handle"), "error in (no error)"=w403) -> ("Reference"=w396:refnum<k15>, "error out"=w402:errorcluster)  [unwired: 7 in, 4 out]
        n149 = call "Pin Name to Reference.vim"("Pin Name"=w398, "type"=refnum<k15> refnum ("instrument handle"), "error in (no error)"=w402) -> ("Reference"=w397:refnum<k15>, "error out"=w389:errorcluster)  [unwired: 7 in, 4 out]
        n150 = for {
          shift-right: [w442] -> w414
          shift-left: w389 -> [w419]
          shift-right: [w440] -> w393
          shift-left: w413 -> [w441]
          tunnel: [w433] -> w412 mode=indexing
          tunnel: [w434] -> w410 mode=indexing
          tunnel: [w435] -> w392 mode=indexing
          tunnel: [w436] -> w411 mode=indexing
          tunnel: w388 -> [w420] mode=indexing
          tunnel: w397 -> [w432]
          tunnel: w396 -> [w431]
          tunnel: w395 -> [w430]
          tunnel: w394 -> [w429]
          tunnel: w391 -> [w422]
          tunnel: w390 -> [w421]
          i -> [w438]
          stop <- w439 stop-if-true
          n151 = call "Set Source.vi"("Set Vin"=w421, "Vin in V"=w420, "error in (no error)"=w419) -> ("error out"=w418:errorcluster)  [unwired: 12 in]
          n152 = call "Stall Data Flow.vim"("value in"=w418, "milliseconds to wait"=w422) -> ("value out"=w423:errorcluster)  [unwired: 1 out]
          n153 = call <instrlib>:"niDCPower Measure Multiple.vi"("error in (no error)"=w423, "instrument handle"=w432) -> ("error out"=w425:errorcluster, "current measurements"=w428:dbl[])  [unwired: 6 in, 2 out]
          n154 = Index Array(array=w428) -> (element=w436:dbl)  [unwired: 1 in]
          n155 = call <instrlib>:"niDCPower Measure Multiple.vi"("error in (no error)"=w425, "instrument handle"=w431) -> ("error out"=w424:errorcluster, "current measurements"=w426:dbl[])  [unwired: 6 in, 2 out]
          n156 = Index Array(array=w426) -> (element=w435:dbl)  [unwired: 1 in]
          n157 = call <instrlib>:"niDMM Read.vi"("error in (no error)"=w424, "instrument handle"=w430) -> ("error out"=w427:errorcluster, "Measurement"=w434:dbl)  [unwired: 7 in, 1 out]
          n158 = call <instrlib>:"niDMM Read.vi"("error in (no error)"=w427, "instrument handle"=w429) -> ("error out"=w437:errorcluster, "Measurement"=w433:dbl)  [unwired: 7 in, 1 out]
          n159 = call <userlib>:"Termination Monitor Status.vi"("Termination Monitor Info in"=w441, "error in (no error)"=w437) -> ("Termination Monitor Info out"=w440:T15, "Terminating?"=w439:bool, "error out"=w442:errorcluster)  [unwired: 11 in]
          "Progress" <- w438
        }
        n160 = Negate(x=w392) -> (-x=w387:dbl[])
        n161 = Bundle By Name(cluster=w417, "Termination Monitor Info"=w393, "Test Results.Input Current in A"=w411, "Test Results.Load Current in A"=w387, "Test Results.Input Voltage in V"=w410, "Test Results.Output Voltage in V"=w412) -> (w416:T16)
      }
      frame "Test: Cleanup DCPower" {
        n162 = Unbundle By Name(w460) -> ("Test Pins.Set Input Voltage"=w455:string, "Test Pins.Set Load Current"=w457:string)
        n163 = call "Pin Name to Reference.vim"("Pin Name"=w457, "type"=refnum<k15> refnum ("instrument handle"), "error in (no error)"=w458) -> ("Reference"=w449:refnum<k15>, "error out"=w448:errorcluster)  [unwired: 7 in, 4 out]
        n164 = call <instrlib>:"niDCPower Configure Output Enabled.vi"("error in (no error)"=w448, "output enabled"=FALSE, "instrument handle"=w449) -> ("error out"=w447:errorcluster, "instrument handle out"=w445:refnum<k15>)  [unwired: 7 in]
        n165 = call <instrlib>:"niDCPower Abort With Channels.vi"("error in (no error)"=w447, "instrument handle"=w445) -> ("error out"=w446:errorcluster)  [unwired: 8 in, 1 out]
        n166 = call "Pin Name to Reference.vim"("Pin Name"=w455, "type"=refnum<k15> refnum ("instrument handle"), "error in (no error)"=w446) -> ("Reference"=w452:refnum<k15>, "error out"=w451:errorcluster)  [unwired: 7 in, 4 out]
        n167 = call <instrlib>:"niDCPower Configure Output Enabled.vi"("error in (no error)"=w451, "output enabled"=FALSE, "instrument handle"=w452) -> ("error out"=w450:errorcluster, "instrument handle out"=w443:refnum<k15>)  [unwired: 7 in]
        n168 = call <instrlib>:"niDCPower Abort With Channels.vi"("error in (no error)"=w450, "instrument handle"=w443) -> ("error out"=w444:errorcluster)  [unwired: 8 in, 1 out]
      }
      frame "Test: Cleanup DMM" {
        n169 = Unbundle By Name(w473) -> ("Test Pins.Measure Input Voltage"=w468:string, "Test Pins.Measure Output Voltage"=w470:string)
        n170 = call "Pin Name to Reference.vim"("Pin Name"=w470, "type"=refnum<k15> refnum ("instrument handle"), "error in (no error)"=w471) -> ("Reference"=w464:refnum<k15>, "error out"=w466:errorcluster)  [unwired: 7 in, 4 out]
        n171 = call <instrlib>:"niDMM Abort.vi"("error in (no error)"=w466, "instrument handle"=w464) -> ("error out"=w465:errorcluster)  [unwired: 8 in, 1 out]
        n172 = call "Pin Name to Reference.vim"("Pin Name"=w468, "type"=refnum<k15> refnum ("instrument handle"), "error in (no error)"=w465) -> ("Reference"=w462:refnum<k15>, "error out"=w467:errorcluster)  [unwired: 7 in, 4 out]
        n173 = call <instrlib>:"niDMM Abort.vi"("error in (no error)"=w467, "instrument handle"=w462) -> ("error out"=w463:errorcluster)  [unwired: 8 in, 1 out]
      }
      frame "Test: Calculate Load" {
        # "Percentage conversion"
        n174 = Unbundle By Name(w490) -> ("Test Results.Output Voltage in V"=w485:dbl[], "Test Results.Input Voltage in V"=w480:dbl[], "Test Inputs.Nominal Output Voltage in V"=w476:dbl)
        n175 = Array Max & Min(array=w485) -> (max value=w487:dbl, min value=w483:dbl)  [unwired: 2 out]
        n176 = Array Max & Min(array=w480) -> (max value=w481:dbl, min value=w482:dbl)  [unwired: 2 out]
        n177 = Subtract(x=w487, y=w483) -> (x-y=w484:dbl)
        n178 = Subtract(x=w481, y=w482) -> (x-y=w479:dbl)
        n179 = Divide(x=w484, y=w479) -> (x/y=w478:dbl)
        n180 = Multiply(x=w478, y=100.0) -> (x*y=w477:dbl)
        n181 = Divide(x=w477, y=w476) -> (x/y=w475:dbl)
        n182 = Bundle By Name(cluster=w490, "Test Results.Line Regulation in %"=w477, "Test Results.Line Regulation in %/V"=w475) -> (w489:T16)
      }
      frame "Test: Update UI" {
        # "If you want to update more indicators in the front panel do it here. It is efficient to update the UI in one case rather than in several cases. Also, it is a good practice to store the results in the data cluster in an efficient format and then get the data from data cluster and update the UI, in that way we could have the front panel independent of how we manipulate the data."
        n183 = Unbundle By Name(w499) -> ("Test Results.Input Voltage in V"=w497:dbl[], "Test Results"=w496:T11, "Test Results.Line Regulation in %/V"=→"Line Regulation (%/V)":dbl, "Test Results.Line Regulation in %"=→"Line Regulation (%)":dbl)
        "Test Results" <- w496
        n184 = Unbundle By Name(w496) -> ("Output Voltage in V"=w495:dbl[])
        n185 = Bundle("Input Voltage in V"=w497, "Output Voltage in V"=w495) -> (→"Line Regulation":T19)  [unwired: 1 in]
      }
      frame "Test: End" {
        # "End of the Test Procedure. Do cleanup of resources or references."
        n186 = property on="Run" class="Bool (strict)"(error in=w506, "Value"=FALSE ("Run"), "DisabledEnum"=T17."Enabled" ("Disabled")) -> (error out=w509:errorcluster)  [unwired: 1 in, 1 out]
        n187 = property on="Terminate" class="Bool (strict)"(error in=w509, "DisabledEnum"=T17."Disabled and Grayed Out" ("Disabled")) -> (error out=w504:errorcluster)  [unwired: 1 in, 1 out]
        n188 = property on="Progress" class="Slide (strict)"(error in=w504, "Visible"=FALSE, "Value"=0 ("Progress")) -> (error out=w503:errorcluster)  [unwired: 1 in, 1 out]
      }
      frame "---------------------Misc-----------------------" {
      }
      frame "Error" {
        # "Handle the error and make sure to clear the error."
        n189 = Unbundle By Name(w518) -> ("Termination Monitor Info.Caller Information.Mode"=w517:T9)
        n190 = case shown="\"MeasurementSuite\"" w517 {
          tunnel: w521 -> [w525 w530 w532]
          tunnel: [w523 w527 w531] -> w519
          tunnel: [_ TRUE _] -> w516
          tunnel: w515 -> [_ w528 _]
          frame "Standalone" {
            w522 = T20 2 items=["no dialog", "OK message", "continue or stop message", "OK message + warnings", "continue/stop + warnings"] ("type of dialog (OK msg:1)")
            n191 = call <vilib>:"General Error Handler.vi"("type of dialog (OK msg:1)"=w522, "error in (no error)"=w525) -> ("error out"=w524:errorcluster)  [unwired: 9 in, 4 out]
            n192 = call <vilib>:"Clear Errors.vi"("error in (no error)"=w524) -> ("error out"=w523:errorcluster)  [unwired: 5 in, 1 out]
          }
          frame "Automation" {
            n193 = call <userlib>:"Release.vi"("Queue in"=w528) -> ("Error Out"=w526:errorcluster)  [unwired: 14 in]
            n194 = Merge Errors(w530, w526) -> (w527:errorcluster)
          }
          frame "MeasurementSuite" {
            n195 = property on="ErrorOccured" class="Clust (strict)"("Val(Sgnl)"=w532) -> (error out=w531:errorcluster)  [unwired: 2 in, 1 out]
          }
        }
      }
      frame "Exit" {
        # "Last case called before stopping the execution. \nError occured in this state will not be captured by Error state."
        n196 = call <userlib>:"Release.vi"("Queue in"=w538, "Error In"=w539) -> ("Error Out"=w534:errorcluster)  [unwired: 13 in]
        n197 = property on="Progress" class="Slide (strict)"(error in=w534, "Visible"=TRUE) -> (error out=w533:errorcluster)  [unwired: 1 in, 1 out]
      }
    }
  }
  "error out" <- w4
  "Header" <- "Line Regulation" ("Header")
